vi "15-FindShortestPath.vi"(4 "Final Position":cluster{"Row":i32, "Col":i32}, 5 "Risk Relief":refnum<vi>, 6 "Initial Position":cluster{"Row":i32, "Col":i32}, 7 "Min Path Risk Relief":refnum<vi>, 8 "Min Risk Array in":i32[][](array[numeric]), 9 "Visited Array in":bool[][](array[boolean]), 10 "map in":T1(c390), 11 "Risk Array in":u8[][](array[numeric])) -> (0 "Min Risk Array out":i32[][](array[numeric]), 1 "Visited Array out":bool[][](array[boolean]), 2 "map out":T1(c390), 3 "Risk Array out":u8[][](array[numeric]))   [LabVIEW 2019, in "15.lvlib"]
uses:
  15.lvlib
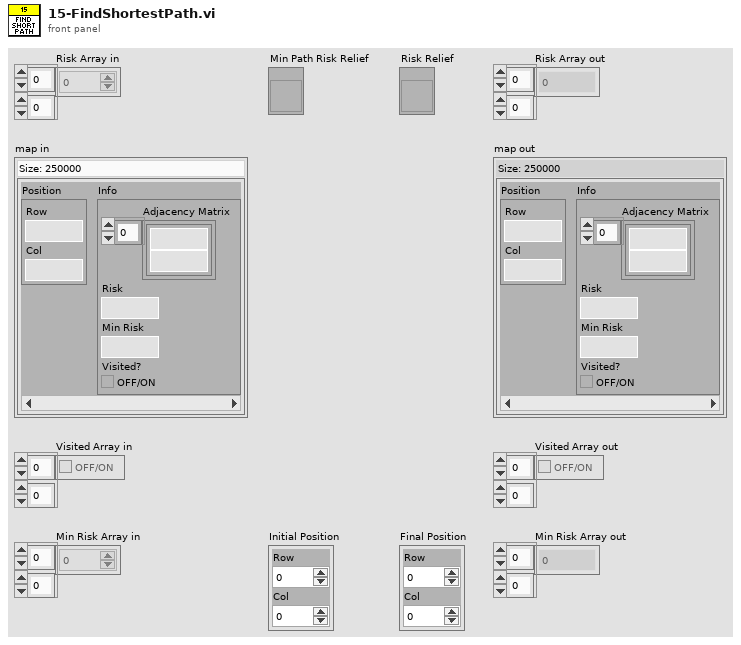
[diagram p1: front panel]
types:
  T1 = map{cluster{"Row":i32, "Col":i32}, cluster{"Adjacency Matrix":cluster{i32, i32}[], "Risk":u8, "Min Risk":i32, "Visited?":bool}}
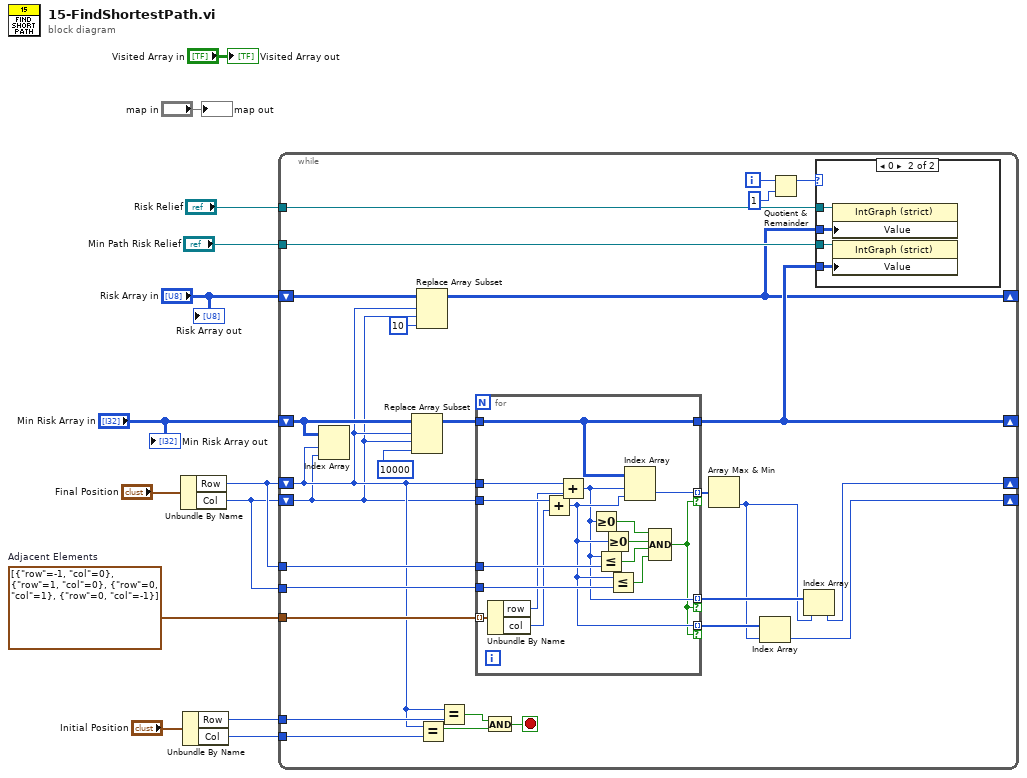
[diagram p0: block diagram]
diagram:
  w5 = cluster{"row":i32, "col":i32}[] [{"row"=-1, "col"=0}, {"row"=1, "col"=0}, {"row"=0, "col"=1}, {"row"=0, "col"=-1}]  # Adjacent Elements
  n1 = Unbundle By Name("Final Position") -> ("Row"=w9:i32, "Col"=w8:i32)
  n2 = Unbundle By Name("Initial Position") -> ("Row"=w6:i32, "Col"=w7:i32)
  n3 = while {
    shift-right: [w24] -> _
    shift-left: "Min Risk Array in" -> [w41]
    shift-right: [w33] -> _
    shift-left: w9 -> [w18]
    shift-right: [w32] -> _
    shift-left: w8 -> [w17]
    tunnel: w5 -> [w38]
    tunnel: w6 -> [w31]
    tunnel: w7 -> [w30]
    tunnel: "Min Path Risk Relief" -> [w23]
    tunnel: w8 -> [w20]
    tunnel: w9 -> [w21]
    shift-right: [w14] -> _
    shift-left: "Risk Array in" -> [w19]
    tunnel: "Risk Relief" -> [w15]
    i -> [w22]
    stop <- w27 stop-if-true
    n4 = Index Array(array=w41, index (row)=w18, index (col)=w17) -> ()  [unwired: 1 out]
    n5 = Replace Array Subset(array=w41, new element=10000 ("new element/subarray"), index (row)=w18, index (col)=w17) -> (w39:i32[][])
    n6 = Replace Array Subset(array=w19, new element=u8 10 ("new element/subarray"), index (row)=w18, index (col)=w17) -> (w14:u8[][])
    n7 = Equal?(x=w18, y=w30) -> (x = y?=w28:bool)
    n8 = Equal?(x=w18, y=w31) -> (x = y?=w29:bool)
    n9 = for {
      tunnel: w39 -> [w58]
      tunnel: w38 -> [w61] mode=indexing
      tunnel: w18 -> [w60]
      tunnel: w17 -> [w59]
      tunnel: [w58] -> w24
      tunnel: [w57] -> w37 mode=indexing if=w46
      tunnel: [w47] -> w36 mode=indexing if=w46
      tunnel: [w49] -> w35 mode=indexing if=w46
      tunnel: w21 -> [w56]
      tunnel: w20 -> [w55]
      n10 = Unbundle By Name(w61) -> ("row"=w48:i32, "col"=w50:i32)
      n11 = Add(x=w59, y=w50) -> (x+y=w49:i32)
      n12 = Add(x=w60, y=w48) -> (x+y=w47:i32)
      n13 = Greater Or Equal To 0?(x=w47) -> (x >= 0?=w54:bool)
      n14 = Less Or Equal?(x=w47, y=w56) -> (x <= y?=w52:bool)
      n15 = Greater Or Equal To 0?(x=w49) -> (x >= 0?=w53:bool)
      n16 = Less Or Equal?(x=w49, y=w55) -> (x <= y?=w51:bool)
      n17 = Index Array(array=w58, index (row)=w47, index (col)=w49) -> (element=w57:i32)
      n18 = Compound Arithmetic op=AND(w54, w53, w52, w51) -> (w46:bool)
    }
    n19 = And(x=w29, y=w28) -> (x .and. y?=w27:bool)
    n20 = Array Max & Min(array=w37) -> (min index (indices)=w34:i32)  [unwired: 3 out]
    n21 = Index Array(array=w35, index=w34) -> (element=w32:i32)
    n22 = Quotient & Remainder(x=w22, y=1) -> (x-y*floor(x/y)=w25:i32)  [unwired: 1 out]
    n23 = Index Array(array=w36, index=w34) -> (element=w33:i32)
    n24 = case shown="0" w25 {
      tunnel: w23 -> [_ w45]
      tunnel: w24 -> [_ w44]
      tunnel: w15 -> [_ w43]
      tunnel: w14 -> [_ w42]
      frame Default {
      }
      frame 0 {
        n25 = property class="IntGraph (strict)"(reference=w43, "Value"=w42) -> ()  [unwired: 1 in, 2 out]
        n26 = property class="IntGraph (strict)"(reference=w45, "Value"=w44) -> ()  [unwired: 1 in, 2 out]
      }
    }
  }
  "map out" <- "map in"
  "Min Risk Array out" <- "Min Risk Array in"
  "Risk Array out" <- "Risk Array in"
  "Visited Array out" <- "Visited Array in"
